vi "Write to Connection.vi"(8 "error in (no error)":errorcluster, 10 "Data to Write":string, 11 "Connection Reference In":refnum<data-value>) -> (0 "error out":errorcluster, 3 "Connection Reference Out":refnum<data-value>)   [LabVIEW 2019, in "Connection Reference.lvlib" / "Connection Reference.lvclass"]
uses:
  <vilib>/gpm_packages/@cs/Network-interface/Source/Connection Reference/Connection Reference/Connection Reference.lvclass
  <vilib>/gpm_packages/@cs/Network-interface/Source/Connection Reference/Connection Reference/Connection Reference.lvclass/Connection Reference.ctl
  <vilib>/gpm_packages/@cs/Network-interface/Source/Connection Reference/IConnection/IConnection.lvclass
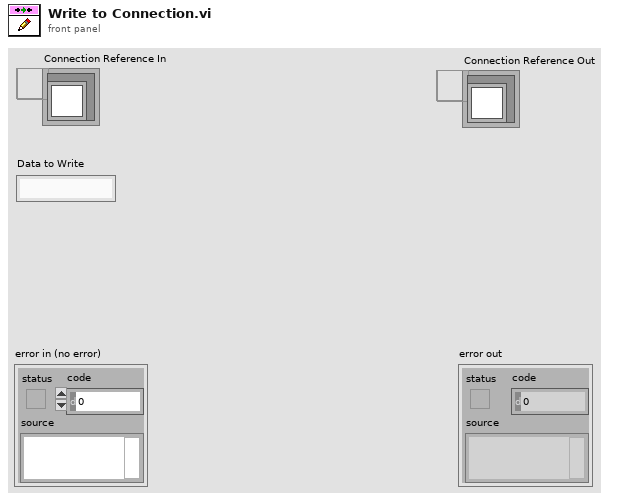
[diagram p1: front panel]
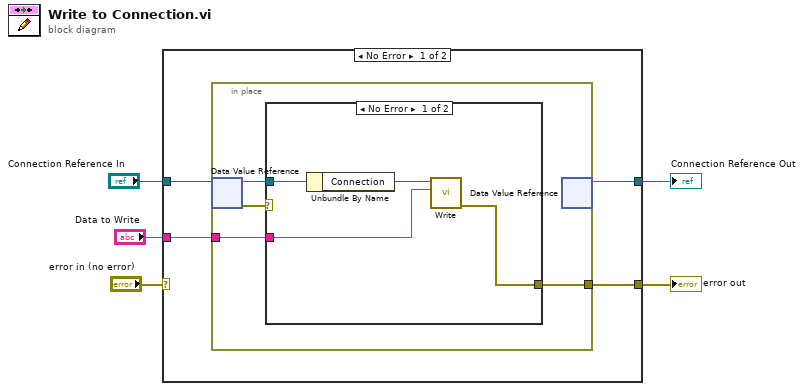
[diagram p0: block diagram]
diagram:
  n1 = case shown="No Error" "error in (no error)" {
    selector: "error in (no error)" -> [_ w19]
    tunnel: "Connection Reference In" -> [w9 w20]
    tunnel: [w8 w20] -> w4
    tunnel: [w7 w19] -> w2
    tunnel: "Data to Write" -> [w6 _]
    frame No Error {
      n2 = in-place {
        in-place-border: [w11] -> w7
        in-place-border: w6 -> [w10]
        n3 = in-place-dvr #1(w9) -> (w13:refnum<class "Connection Reference.lvclass">, w12:errorcluster)
        n4 = case shown="No Error" w12 {
          selector: w12 -> [_ w18]
          tunnel: w13 -> [w17 _]
          tunnel: [w16 w18] -> w11
          tunnel: w10 -> [w15 _]
          frame No Error {
            n5 = Unbundle By Name(w17) -> ("Connection"=w14:refnum<class "IConnection.lvclass">)
            n6 = call-dynamic "Write.vi"("Data to Write"=w15, "IConnection in"=w14) -> ("error out"=w16:errorcluster)  [unwired: 8 in, 1 out]
          }
          frame Error {
            # "#todo add useful error here"
          }
        }
        n7 = in-place-dvr #1() -> (w8:refnum<data-value>)  [unwired: 1 in, 1 out]
      }
    }
    frame Error {
    }
  }
  "error out" <- w2
  "Connection Reference Out" <- w4
